vi "Pix2U32.vi"(10 "input cluster":T1) -> (1 "pixmap":u32[](array[numeric]))   [LabVIEW 2022 SP3]
doc: "This VI follows the VI \"Read PNG File\" and gets its outer cluster as an entry. From that it uses the VI \"Unflatten Pixmap\" to create a 2D array containing the pixels of the image that has been read. From that it reshapes the 2D array in a 1D array adding the length and the height respectively at first and second index. Finnally it gives back this 1D array (U32).\n\nInput :\n- The cluster coming from the VI \"Read PNG File\"\n\nOutput :\n- A 1D array containing the length, the height and the pixmap (U32)"
uses:
  <vilib>/picture/picture.llb/imagedata.ctl
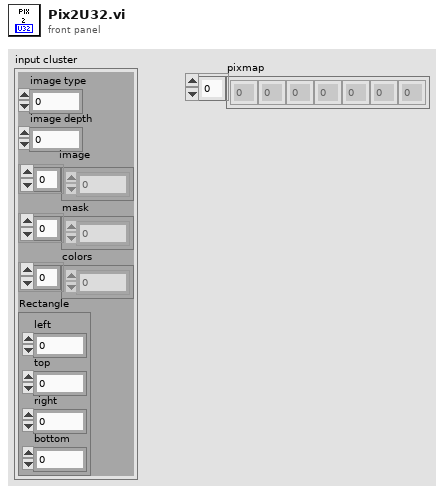
[diagram p1: front panel]
types:
  T1 = typedef "imagedata.ctl" = cluster{"image type":i32, "image depth":i32, "image":u8[], "mask":u8[], "colors":u32[], "Rectangle":cluster{"left":i16, "top":i16, "right":i16, "bottom":i16}}
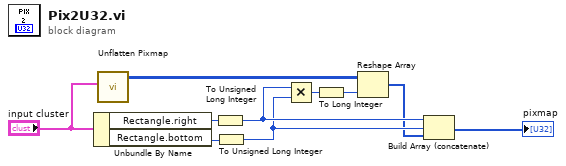
[diagram p0: block diagram]
diagram:
  n1 = Unbundle By Name("input cluster") -> ("Rectangle.right"=w2:i16, "Rectangle.bottom"=w3:i16)
  n2 = call <vilib>:"Unflatten Pixmap.vi"("image data"="input cluster") -> ("24-bit pixmap"=w7:u32[][])  [unwired: 4 in, 6 out]
  n3 = To Unsigned Long Integer(number=w2) -> (unsigned 32bit integer=w10:u32)
  n4 = To Unsigned Long Integer(number=w3) -> (unsigned 32bit integer=w6:u32)
  n5 = Multiply(x=w10, y=w6) -> (x*y=w4:u32)
  n6 = To Long Integer(number=w4) -> (32bit integer=w8:i32)
  n7 = Reshape Array(w7, w8) -> (w5:u32[])
  n8 = Build Array (concatenate) "Build Array"(w10, w6, w5) -> (→"pixmap":u32[])
